vi "Configuration_table.vi"(11 "Configuration Queue":refnum<queue>) -> ()   [LabVIEW 2013, in "main.lvlib"]
uses:
  main.lvlib
  Controls/Reference AE Control.ctl
  Controls/Reference Cluster.ctl
  Bluetooth/MessageStructure.ctl
panel:
  in  "ActivityBox":bool caption="Efter stimulering"
  out "SegmentNumberString":string caption="Nummer"
  out "UndersøgelsesString":string caption="Undersøgelse"
  in  "ListboxLeftSegmentNr":i32(listbox) caption="Venstre"
  in  "ListboxRightSegmentNr":i32(listbox) caption="Højre"
  in  "ListboxMeasurementArea":i32(listbox) caption="Segment"
  in  "ListboxMeasurementTechnique":i32(listbox) caption="Teknik"
  in  "ListboxMeasurementMeth":i32(listbox) caption="Metode"
  out "Left Time Table":string[][](table)
  out "LeftArmPressureTable":string[][](table)
  out "LeftArmPulsTable":string[][](table)
  out "Right Time Table":string[][](table)
  out "RightArmPressureTable":string[][](table)
  out "RightArmPulsTable":string[][](table)
  in  "EditPressureBtn":bool
  in  "AddNewMeasurementBtn":bool
  in  "HeightAdjustmentInt":dbl caption="Højdejustering"
  in  "PalpationLeft":string(combo)="None" caption="Palpation"
  in  "PalpationRight":string(combo)="None" caption="Palpation"
  in  "Stop":bool
  # "Venstre"
  # "Sys"
  # "Dia"
  # "Puls"
  # "Tid"
  # "Højre"
  # "Tid"
  # "Sys"
  # "Dia"
  # "Puls"
  # "Palpation"
  # "cm"
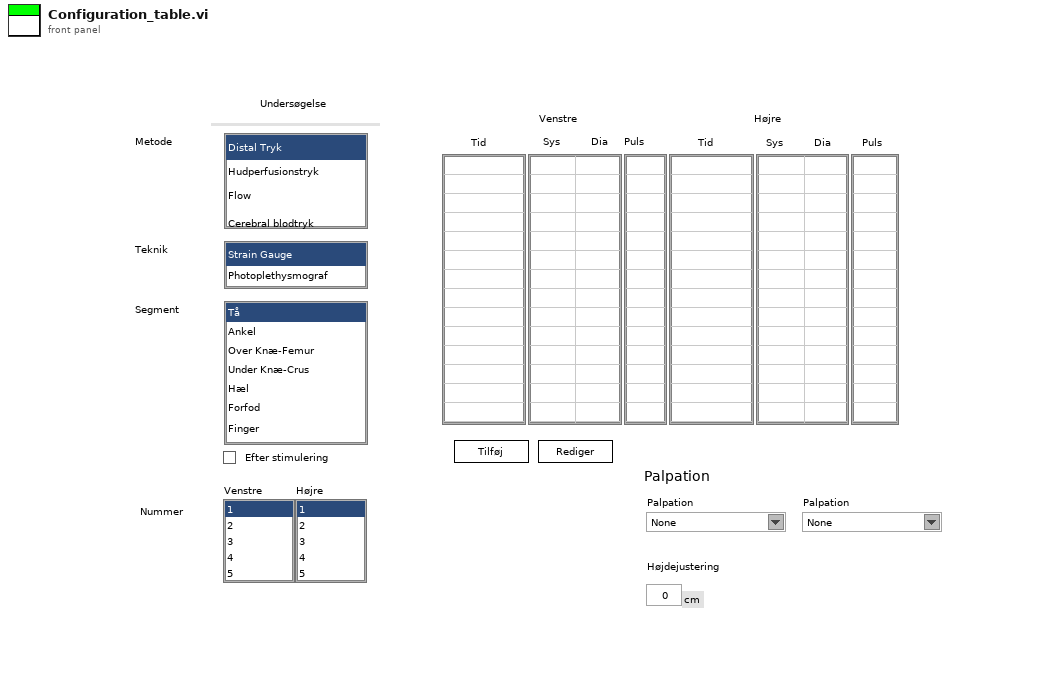
[diagram p1: front panel]
types:
  T1 = cluster{"sys":dbl, "dia":dbl, "puls":dbl, "date":string, "time":string, "code":string, "serial":string, "temp":dbl, "activity":string}
  T2 = typedef "main.lvlib/Reference AE Control.ctl" = enum16{"Initialize", "Set Menu", "Set Profile", "Set Configuration", "Set Configuration_old", "Set Configuration_new", "Set Configuration Method", "Set Acquisition", "Set Data", "Set Journal", "Get"}
  T3 = typedef "main.lvlib/Reference Cluster.ctl" = cluster{"Menu":cluster{"References":cluster{"Stop Acq":refnum<vi>, "MenuExit":refnum<vi>, "MenuStartADC":refnum<vi>, "PersonalInfoString":refnum<vi>, "Profile":refnum<vi>, "Configuration":refnum<vi>, "Acquisition":refnum<vi>, "Data":refnum<vi>, "Journal":refnum<vi>}}, "Profile":cluster{"References":cluster{"Search Patient ID":refnum<vi>, "Name":refnum<vi>, "CommentStr":refnum<vi>, "Listbox Patient ID":refnum<vi>, "ListboxDoctor":refnum<vi>, "ListboxOperator":refnum<vi>, "HospitalName":refnum<vi>, "HospitalDepartment":refnum<vi>, "HospitalAddress":refnum<vi>, "EditHospInfo":refnum<vi>, "Add Patient ID Btn":refnum<vi>, "Query Worklist":refnum<vi>}}, "Configuration":cluster{"References":cluster{"ListboxMeasurementArea":refnum<vi>, "ListboxMeasurementTechnique":refnum<vi>, "ListboxMeasurementMeth":refnum<vi>, "ListboxRightSegmentNr":refnum<vi>, "ListboxLeftSegmentNr":refnum<vi>, "HeightAdjustmentInt":refnum<vi>, "PalpationRight":refnum<vi>, "PalpationLeft":refnum<vi>, "ActivityBox":refnum<vi>}, "New method":cluster{"AddNewMeasurementBtn":refnum<vi>, "Left Time Table":refnum<vi>, "Right Time Table":refnum<vi>}, "Old method":cluster{"LeftArmPressureTable":refnum<vi>, "RightArmPressureTable":refnum<vi>, "SaveArmPressureBtn":refnum<vi>, "Puls":refnum<vi>, "TempTwo":refnum<vi>, "TempOne":refnum<vi>}, "Method":string}, "Acquisition":cluster{"References":cluster{"SegmentAcqString":refnum<vi>, "RingActGraph":refnum<vi>}}, "Data":cluster{"References":cluster{"cmString":refnum<vi>, "AdjustedHeight":refnum<vi>, "Menu":refnum<vi>, "Tangent On/Off":refnum<vi>, "FilterControl":refnum<vi>}}, "Journal":cluster{"References":cluster{"ReportSelection":refnum<vi>, "Data":refnum<vi>, "GenerateReport":refnum<vi>, "Menu":refnum<vi>, "Send To PACS":refnum<vi>}}}
  T4 = cluster{"ListboxMeasurementArea":refnum<vi>, "ListboxMeasurementTechnique":refnum<vi>, "ListboxMeasurementMeth":refnum<vi>, "ListboxRightSegmentNr":refnum<vi>, "ListboxLeftSegmentNr":refnum<vi>, "HeightAdjustmentInt":refnum<vi>, "PalpationRight":refnum<vi>, "PalpationLeft":refnum<vi>, "ActivityBox":refnum<vi>}
  T5 = typedef "LVRectTypeDef.ctl" = cluster{"Left":i16, "Top":i16, "Right":i16, "Bottom":i16}
  T6 = cluster{"ArmPressureSys":dbl, "ArmPressureDia":dbl, "ArmPuls":dbl, "Side":string}
  T7 = typedef "main.lvlib/MessageStructure.ctl" = cluster{"Type":i32, "Device type":i32, "Date":string, "Time":string, "Serial Number":string, "Sys":i32, "Dia":i32, "Puls":i32, "MAP":i32, "Code":string}
  T8 = cluster{"data":cluster{"sys":dbl, "dia":dbl, "puls":dbl, "date":string, "time":string, "code":string, "serial":string, "temp":dbl, "activity":string}, "Side":string}
  T9 = cluster{"sys":dbl, "dia":dbl, "puls":dbl, "date":string, "time":string, "code":string, "serial":string, "temp":dbl, "activity":string}[]
  T10 = cluster{"data":cluster{"sys":dbl, "dia":dbl, "puls":dbl, "date":string, "time":string, "code":string, "serial":string, "temp":dbl, "activity":string}, string}
  T11 = cluster{"AddNewMeasurementBtn":refnum<vi>, "Left Time Table":refnum<vi>, "Right Time Table":refnum<vi>}
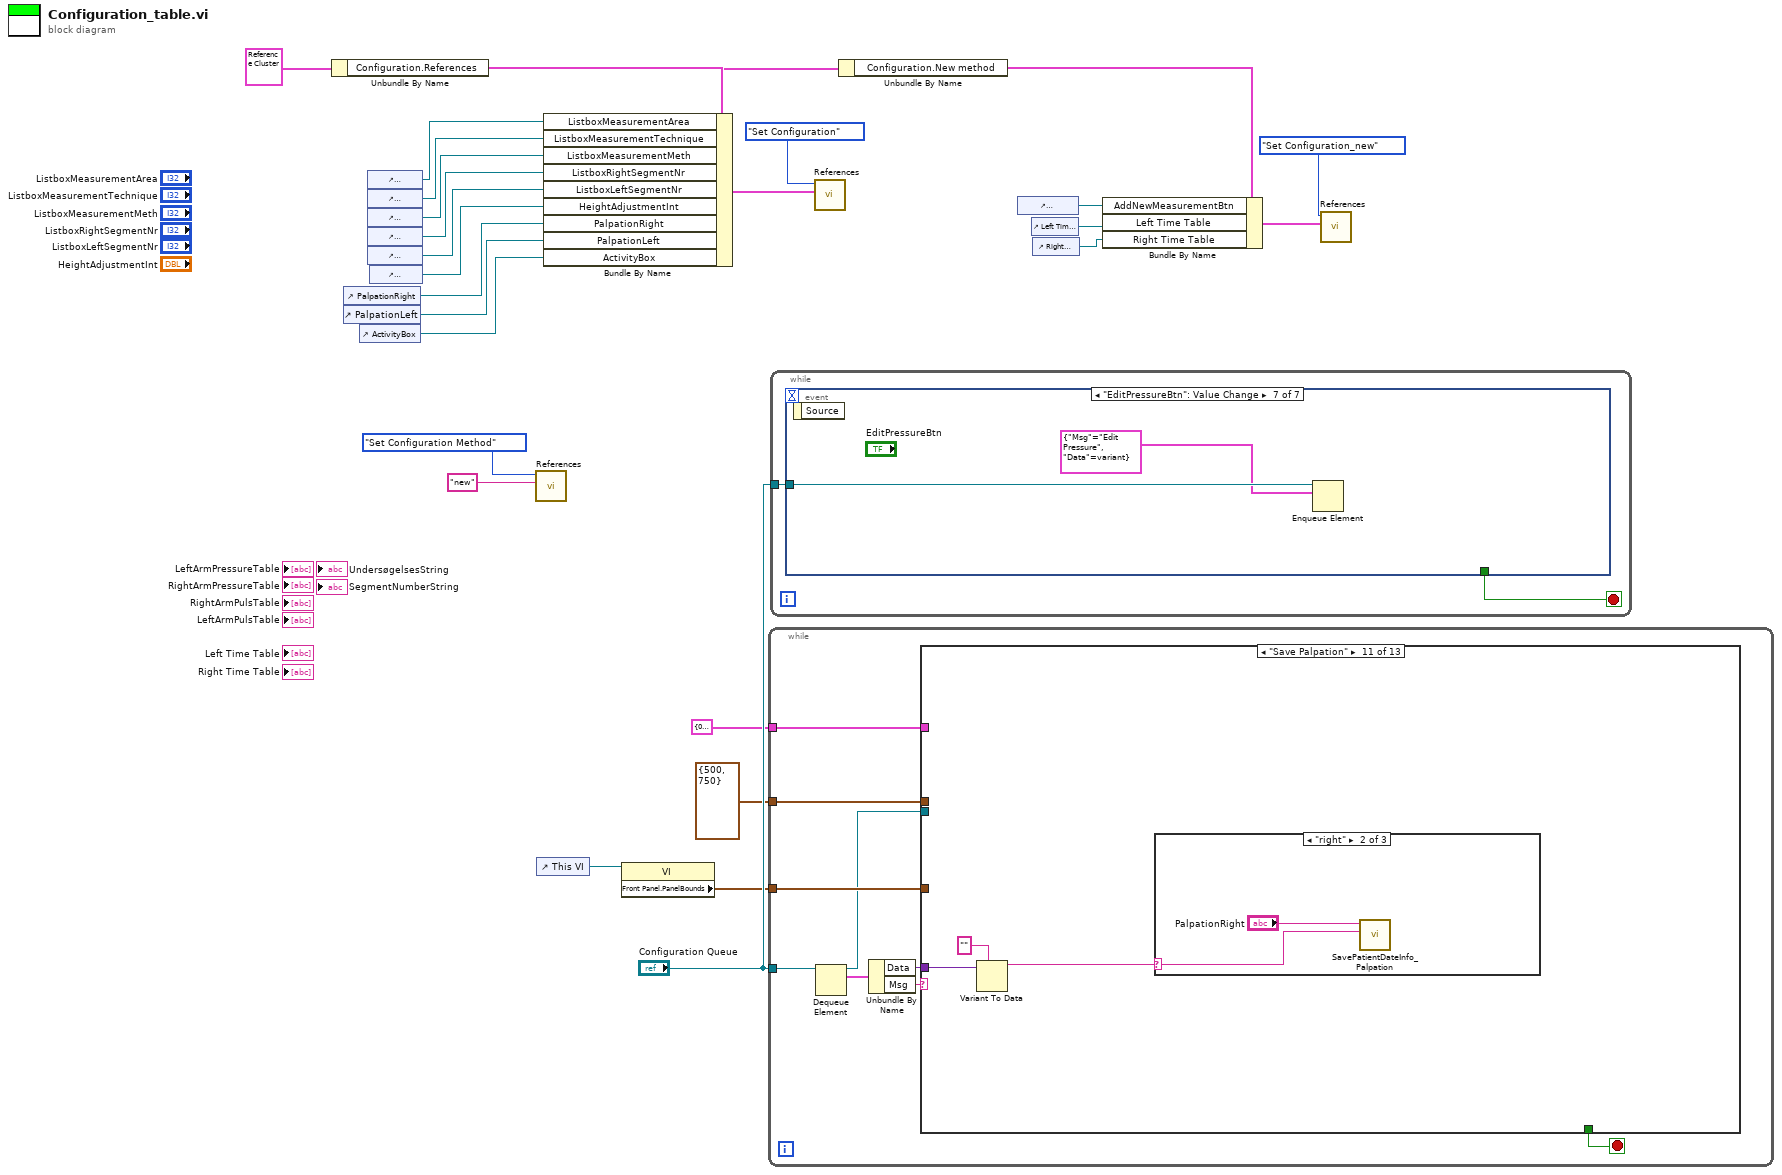
[diagram p0: block diagram]
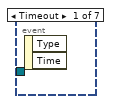
[diagram p2: hidden frame]
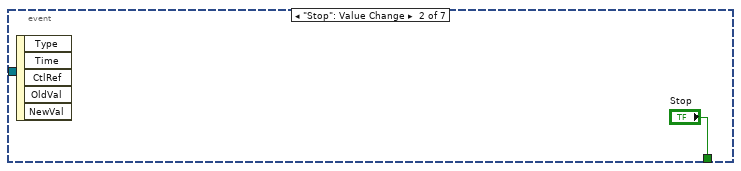
[diagram p3: hidden frame]
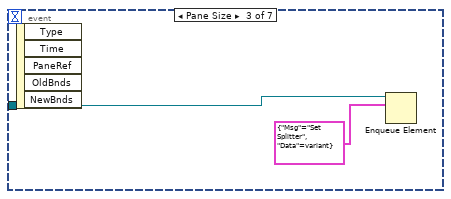
[diagram p4: hidden frame]
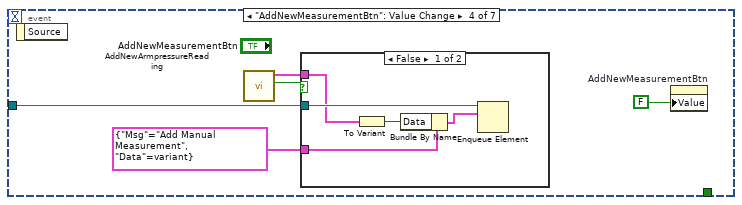
[diagram p5: hidden frame]
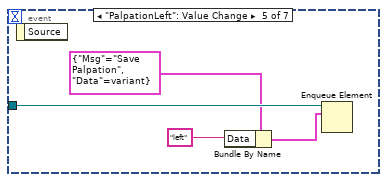
[diagram p7: hidden frame]
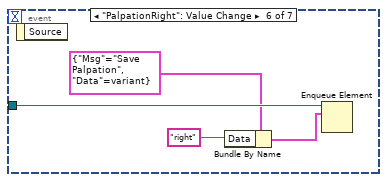
[diagram p8: hidden frame]
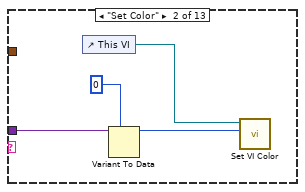
[diagram p10: hidden frame]
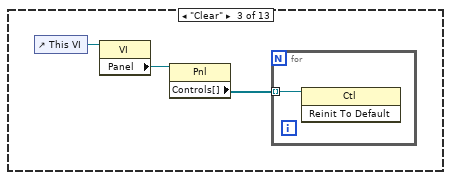
[diagram p11: hidden frame]
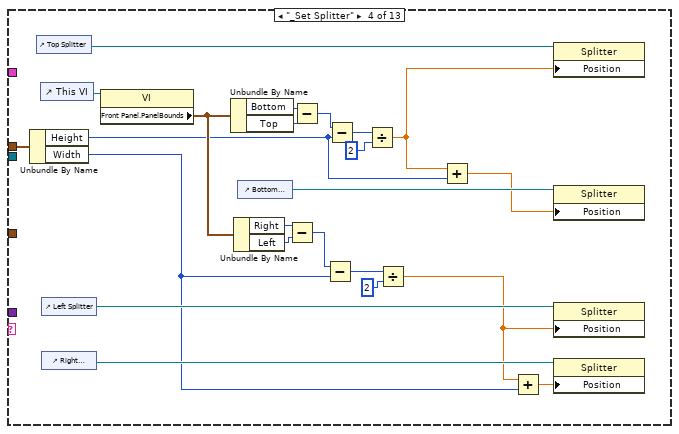
[diagram p12: hidden frame]
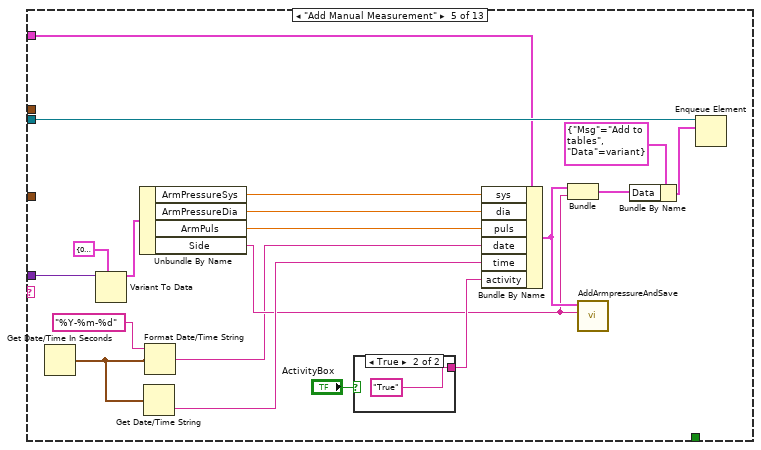
[diagram p13: hidden frame]
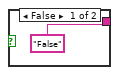
[diagram p14: hidden frame]
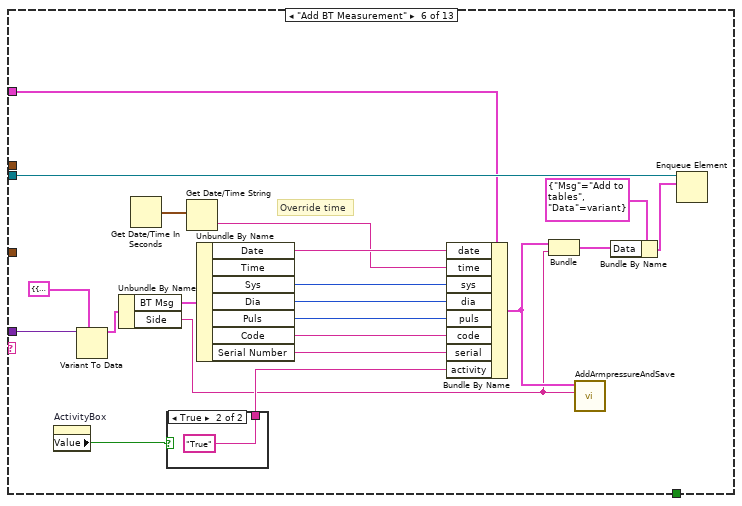
[diagram p15: hidden frame]
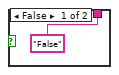
[diagram p16: hidden frame]
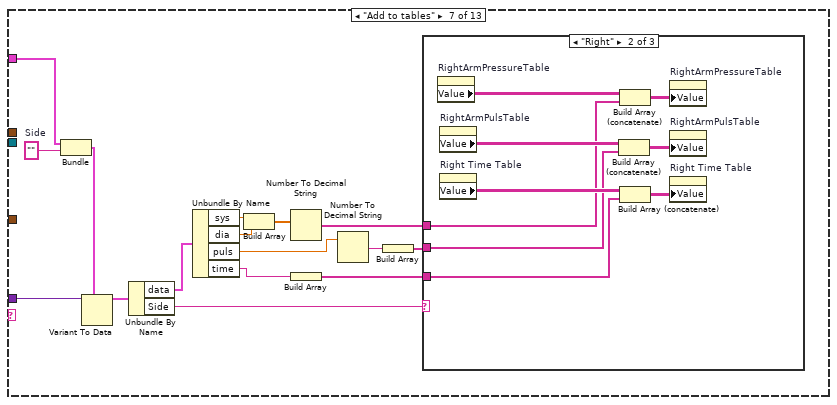
[diagram p17: hidden frame]
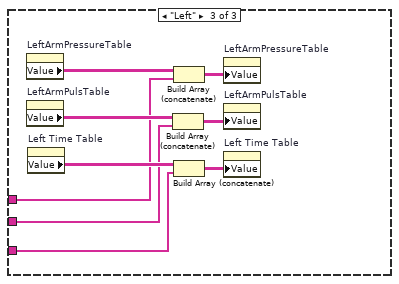
[diagram p19: hidden frame]
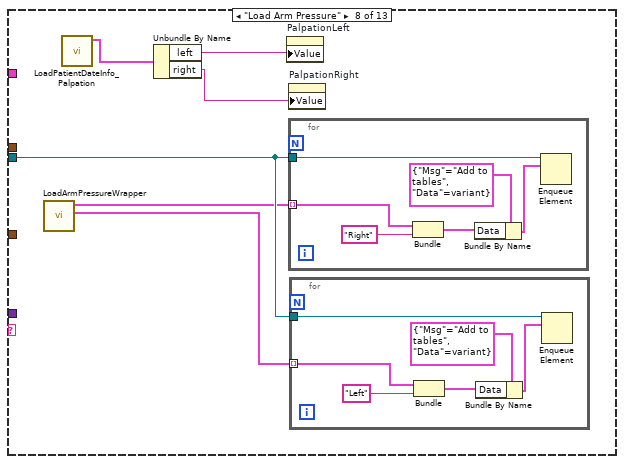
[diagram p20: hidden frame]
diagram:
  w10 = T3 {"Menu"={"References"={"Stop Acq"=refnum, "MenuExit"=refnum, "MenuStartADC"=refnum, "PersonalInfoString"=refnum, "Profile"=refnum, "Configuration"=refnum, "Acquisition"=refnum, "Data"=refnum, "Journal"=refnum}}, "Profile"={"References"={"Search Patient ID"=refnum, "Name"=refnum, "CommentStr"=refnum, "Listbox Patient ID"=refnum, "ListboxDoctor"=refnum, "ListboxOperator"=refnum, "HospitalName"=refnum, "HospitalDepartment"=refnum, "HospitalAddress"=refnum, "EditHospInfo"=refnum, "Add Patient ID Btn"=refnum, "Query Worklist"=refnum}}, "Configuration"={"References"={"ListboxMeasurementArea"=refnum, "ListboxMeasurementTechnique"=refnum, "ListboxMeasurementMeth"=refnum, "ListboxRightSegmentNr"=refnum, "ListboxLeftSegmentNr"=refnum, "HeightAdjustmentInt"=refnum, "PalpationRight"=refnum, "PalpationLeft"=refnum, "ActivityBox"=refnum}, "New method"={"AddNewMeasurementBtn"=refnum, "Left Time Table"=refnum, "Right Time Table"=refnum}, "Old method"={"LeftArmPressureTable"=refnum, "RightArmPressureTable"=refnum, "SaveArmPressureBtn"=refnum, "Puls"=refnum, "TempTwo"=refnum, "TempOne"=refnum}, "Method"=""}, "Acquisition"={"References"={"SegmentAcqString"=refnum, "RingActGraph"=refnum}}, "Data"={"References"={"cmString"=refnum, "AdjustedHeight"=refnum, "Menu"=refnum, "Tangent On/Off"=refnum, "FilterControl"=refnum}}, "Journal"={"References"={"ReportSelection"=refnum, "Data"=refnum, "GenerateReport"=refnum, "Menu"=refnum, "Send To PACS"=refnum}}}
  n1 = Unbundle By Name(w10) -> ("Configuration.References"=w11:T4)
  n2 = control-ref of="PalpationRight"() -> (w14:refnum<vi>)
  n3 = control-ref of="PalpationLeft"() -> (w13:refnum<vi>)
  n4 = control-ref of="ActivityBox"() -> (w12:refnum<vi>)
  n5 = control-ref of="ListboxMeasurementArea"() -> (w26:refnum<vi>)
  n6 = control-ref of="ListboxMeasurementTechnique"() -> (w25:refnum<vi>)
  n7 = control-ref of="ListboxMeasurementMeth"() -> (w24:refnum<vi>)
  n8 = control-ref of="ListboxRightSegmentNr"() -> (w23:refnum<vi>)
  n9 = control-ref of="ListboxLeftSegmentNr"() -> (w22:refnum<vi>)
  n10 = control-ref of="HeightAdjustmentInt"() -> (w21:refnum<vi>)
  n11 = call "References.vi"("variant"="new", "Reference AE Control"=Reference_AE_Control."Set Configuration Method") -> ()  [unwired: 8 in, 2 out]
  n12 = control-ref of="This VI"() -> (w17:refnum<vi>)
  n13 = Bundle By Name(cluster=w11, "ListboxMeasurementArea"=w26, "ListboxMeasurementTechnique"=w25, "ListboxMeasurementMeth"=w24, "ListboxRightSegmentNr"=w23, "ListboxLeftSegmentNr"=w22, "HeightAdjustmentInt"=w21, "PalpationRight"=w14, "PalpationLeft"=w13, "ActivityBox"=w12) -> (w19:T4)
  n14 = property class="VI"(reference=w17) -> ("Front Panel.PanelBounds"=w16:T5)  [unwired: 1 in, 2 out]
  n15 = while {
    tunnel: "Configuration Queue" -> [w35]
    tunnel: cluster{"Height":i32, "Width":i32} {"Height"=500, "Width"=750} -> [w30]
    tunnel: w16 -> [w29]
    tunnel: T1 {"sys"=0.0, "dia"=0.0, "puls"=0.0, "date"="", "time"="", "code"="", "serial"="", "temp"=0.0, "activity"=""} ("data") -> [w27]
    stop <- w32 stop-if-true
    n16 = Dequeue Element(queue=w35) -> (queue out=w28:refnum<queue>, element=w34:cluster{"Msg":string, "Data":variant})  [unwired: 2 in, 2 out]
    n17 = Unbundle By Name(w34) -> ("Data"=w31:variant, "Msg"=w33:string)
    n18 = case shown="\"Save Palpation\"" w33 {
      tunnel: [_ _ _ _ _ _ _ _ _ _ _ w185 w207] -> w32
      tunnel: w31 -> [_ w36 _ _ w85 w108 w126 _ _ _ w179 _ _]
      tunnel: w30 -> [_ _ _ w52 _ _ _ _ _ _ _ w194 _]
      tunnel: w29 -> [_ _ _ _ _ _ _ _ _ _ _ w184 _]
      tunnel: w28 -> [_ _ _ _ w81 w106 _ w150 w163 _ _ _ _]
      tunnel: w27 -> [_ _ _ _ w76 w93 w122 _ _ _ _ _ _]
      frame "", Default {
      }
      frame "Set Color" {
        n19 = control-ref of="This VI"() -> (w39:refnum<vi>)
        n20 = Variant To Data(type=u32 0 ("Pane Color"), Variant=w36) -> (data=w37:u32)  [unwired: 1 in, 1 out]
        n21 = call "Set VI Color.vi"("Pane Color"=w37, "VI in"=w39) -> ()  [unwired: 10 in]
      }
      frame "Clear" {
        n22 = control-ref of="This VI"() -> (w42:refnum<vi>)
        n23 = property class="VI"(reference=w42) -> ("Panel"=w41:refnum<vi>)  [unwired: 1 in, 2 out]
        n24 = property class="Pnl"(reference=w41) -> ("Controls[]"=w40:refnum<vi>[])  [unwired: 1 in, 2 out]
        n25 = for {
          tunnel: w40 -> [w43] mode=indexing
          n26 = invoke class="Ctl" method="Reinit To Default"(reference=w43) -> ()  [unwired: 2 in, 3 out]
        }
      }
      frame "_Set Splitter" {
        n27 = Unbundle By Name(w52) -> ("Height"=w50:i32, "Width"=w45:i32)
        n28 = control-ref of="Top Splitter"() -> (w60:refnum<vi>)
        n29 = control-ref of="This VI"() -> (w66:refnum<vi>)
        n30 = control-ref of="Left Splitter"() -> (w53:refnum<vi>)
        n31 = control-ref of="Right Splitter"() -> (w47:refnum<vi>)
        n32 = property class="VI"(reference=w66) -> ("Front Panel.PanelBounds"=w59:T5)  [unwired: 1 in, 2 out]
        n33 = Unbundle By Name(w59) -> ("Bottom"=w65:i16, "Top"=w64:i16)
        n34 = Unbundle By Name(w59) -> ("Right"=w58:i16, "Left"=w57:i16)
        n35 = control-ref of="Bottom Splitter"() -> (w49:refnum<vi>)
        n36 = Subtract(x=w58, y=w57) -> (x-y=w56:i16)
        n37 = Subtract(x=w65, y=w64) -> (x-y=w63:i16)
        n38 = Subtract(x=w56, y=w45) -> (x-y=w55:i32)
        n39 = Subtract(x=w63, y=w50) -> (x-y=w62:i32)
        n40 = Divide(x=w62, y=2) -> (x/y=w51:dbl)
        n41 = Divide(x=w55, y=u32 2) -> (x/y=w46:dbl)
        n42 = Add(x=w51, y=w50) -> (x+y=w48:dbl)
        n43 = Add(x=w46, y=w45) -> (x+y=w44:dbl)
        n44 = property class="Splitter"(reference=w60, "Position"=w51) -> ()  [unwired: 1 in, 2 out]
        n45 = property class="Splitter"(reference=w49, "Position"=w48) -> ()  [unwired: 1 in, 2 out]
        n46 = property class="Splitter"(reference=w53, "Position"=w46) -> ()  [unwired: 1 in, 2 out]
        n47 = property class="Splitter"(reference=w47, "Position"=w44) -> ()  [unwired: 1 in, 2 out]
      }
      frame "Add Manual Measurement" {
        n48 = Get Date/Time In Seconds() -> (seconds since 1Jan1904=w68:timestamp)
        n49 = Variant To Data(type=T6 {"ArmPressureSys"=0.0, "ArmPressureDia"=0.0, "ArmPuls"=0.0, "Side"=""} ("output cluster"), Variant=w85) -> (data=w74:T6)  [unwired: 1 in, 1 out]
        n50 = Unbundle By Name(w74) -> ("ArmPressureSys"=w73:dbl, "ArmPressureDia"=w72:dbl, "ArmPuls"=w71:dbl, "Side"=w70:string)
        n51 = Get Date/Time String(seconds (now)=w68) -> (time string=w84:string)  [unwired: 2 in, 1 out]
        n52 = Format Date/Time String(time format string (%c)="%Y-%m-%d", seconds (now)=w68) -> (date/time string=w67:string)  [unwired: 1 in]
        n53 = case shown="True" "ActivityBox" {
          tunnel: ["False" "True"] -> w82
          frame False {
          }
          frame True {
          }
        }
        n54 = Bundle By Name(cluster=w76, "sys"=w73, "dia"=w72, "puls"=w71, "date"=w67, "time"=w84, "activity"=w82) -> (w77:T1)
        n55 = Bundle("data"=w77, "Side"=w70) -> (w78:T8)  [unwired: 1 in]
        n56 = call "AddArmpressureAndSave.vi"("Side(Left/Right)"=w70, "data"=w77) -> ()  [unwired: 9 in, 1 out]
        n57 = Bundle By Name(cluster=cluster{"Msg":string, "Data":variant} {"Msg"="Add to tables", "Data"=variant} ("element"), "Data"=w78) -> (w79:cluster{"Msg":string, "Data":variant})
        n58 = Enqueue Element(queue=w81, element=w79) -> ()  [unwired: 2 in, 3 out]
      }
      frame "Add BT Measurement" {
        # "Override time"
        n59 = property on="ActivityBox" class="Bool (strict)"() -> ("Value"=w94:bool)  [unwired: 2 in, 2 out]
        n60 = Variant To Data(type=cluster{"BT Msg":T7, "Side":string} {"BT Msg"={"Type"=0, "Device type"=0, "Date"="", "Time"="", "Serial Number"="", "Sys"=0, "Dia"=0, "Puls"=0, "MAP"=0, "Code"=""}, "Side"=""}, Variant=w108) -> (data=w97:cluster{"BT Msg":T7, "Side":string})  [unwired: 1 in, 1 out]
        n61 = Unbundle By Name(w97) -> ("BT Msg"=w96:T7, "Side"=w95:string)
        n62 = Get Date/Time In Seconds() -> (seconds since 1Jan1904=w89:timestamp)
        n63 = case shown="True" w94 {
          tunnel: ["False" "True"] -> w107
          frame False {
          }
          frame True {
          }
        }
        n64 = Get Date/Time String(seconds (now)=w89) -> (time string=w88:string)  [unwired: 2 in, 1 out]
        n65 = Unbundle By Name(w96) -> ("Date"=w91:string, "Sys"=w92:i32, "Dia"=w101:i32, "Puls"=w100:i32, "Code"=w99:string, "Serial Number"=w98:string)  [unwired: 1 out]
        n66 = Bundle By Name(cluster=w93, "date"=w91, "time"=w88, "sys"=w92, "dia"=w101, "puls"=w100, "code"=w99, "serial"=w98, "activity"=w107) -> (w102:T1)
        n67 = Bundle("data"=w102, "Side"=w95) -> (w103:T8)  [unwired: 1 in]
        n68 = call "AddArmpressureAndSave.vi"("Side(Left/Right)"=w95, "data"=w102) -> ()  [unwired: 9 in, 1 out]
        n69 = Bundle By Name(cluster=cluster{"Msg":string, "Data":variant} {"Msg"="Add to tables", "Data"=variant} ("element"), "Data"=w103) -> (w104:cluster{"Msg":string, "Data":variant})
        n70 = Enqueue Element(queue=w106, element=w104) -> ()  [unwired: 2 in, 3 out]
      }
      frame "Add to tables" {
        w123 = ""  # Side
        n71 = Bundle("data"=w122, "Side"=w123) -> (w121:T8)  [unwired: 1 in]
        n72 = Variant To Data(type=w121, Variant=w126) -> (data=w125:T8)  [unwired: 1 in, 1 out]
        n73 = Unbundle By Name(w125) -> ("data"=w118:T1, "Side"=w124:string)
        n74 = Unbundle By Name(w118) -> ("sys"=w119:dbl, "dia"=w120:dbl, "puls"=w114:dbl, "time"=w111:string)
        n75 = Build Array(w119, w120) -> (w117:dbl[])
        n76 = Number To Decimal String(number=w117) -> (decimal integer string=w116:string[])  [unwired: 1 in]
        n77 = Build Array(w111) -> (w115:string[])
        n78 = Number To Decimal String(number=w114) -> (decimal integer string=w112:string)  [unwired: 1 in]
        n79 = Build Array(w112) -> (w113:string[])
        n80 = case shown="\"Right\"" w124 {
          tunnel: w113 -> [_ w129 w138]
          tunnel: w116 -> [_ w128 w137]
          tunnel: w115 -> [_ w127 w136]
          frame "False", Default {
          }
          frame "Right" {
            n81 = property on="RightArmPressureTable" class="Tbl (strict)"() -> ("Value"=w135:string[][])  [unwired: 2 in, 2 out]
            n82 = property on="RightArmPulsTable" class="Tbl (strict)"() -> ("Value"=w132:string[][])  [unwired: 2 in, 2 out]
            n83 = property on="Right Time Table" class="Tbl (strict)"() -> ("Value"=w131:string[][])  [unwired: 2 in, 2 out]
            n84 = Build Array (concatenate)(w132, w129) -> (w133:string[][])
            n85 = Build Array (concatenate)(w135, w128) -> (w134:string[][])
            n86 = Build Array (concatenate)(w131, w127) -> (w130:string[][])
            n87 = property on="RightArmPressureTable" class="Tbl (strict)"("Value"=w134) -> ()  [unwired: 2 in, 2 out]
            n88 = property on="RightArmPulsTable" class="Tbl (strict)"("Value"=w133) -> ()  [unwired: 2 in, 2 out]
            n89 = property on="Right Time Table" class="Tbl (strict)"("Value"=w130) -> ()  [unwired: 2 in, 2 out]
          }
          frame "Left" {
            n90 = property on="LeftArmPressureTable" class="Tbl (strict)"() -> ("Value"=w144:string[][])  [unwired: 2 in, 2 out]
            n91 = property on="LeftArmPulsTable" class="Tbl (strict)"() -> ("Value"=w143:string[][])  [unwired: 2 in, 2 out]
            n92 = property on="Left Time Table" class="Tbl (strict)"() -> ("Value"=w142:string[][])  [unwired: 2 in, 2 out]
            n93 = Build Array (concatenate)(w143, w138) -> (w140:string[][])
            n94 = Build Array (concatenate)(w144, w137) -> (w141:string[][])
            n95 = Build Array (concatenate)(w142, w136) -> (w139:string[][])
            n96 = property on="LeftArmPressureTable" class="Tbl (strict)"("Value"=w141) -> ()  [unwired: 2 in, 2 out]
            n97 = property on="LeftArmPulsTable" class="Tbl (strict)"("Value"=w140) -> ()  [unwired: 2 in, 2 out]
            n98 = property on="Left Time Table" class="Tbl (strict)"("Value"=w139) -> ()  [unwired: 2 in, 2 out]
          }
        }
      }
      frame "Load Arm Pressure" {
        n99 = call "LoadArmPressureWrapper.vi"() -> ("Armpressure Left"=w145:T9, "Armpressure Right"=w146:T9)  [unwired: 9 in, 1 out]
        n100 = call "LoadPatientDateInfo_Palpation.vi"() -> ("palpation"=w147:cluster{"right":string, "left":string})  [unwired: 10 in, 1 out]
        n101 = Unbundle By Name(w147) -> ("left"=w149:string, "right"=w148:string)
        n102 = property on="PalpationLeft" class="CmbBox"("Value"=w149) -> ()  [unwired: 2 in, 2 out]
        n103 = property on="PalpationRight" class="CmbBox"("Value"=w148) -> ()  [unwired: 2 in, 2 out]
        n104 = for {
          tunnel: w150 -> [w159]
          tunnel: w146 -> [w158] mode=indexing
          n105 = Bundle("data"=w158, "Right") -> (w160:T10)  [unwired: 1 in]
          n106 = Bundle By Name(cluster=cluster{"Msg":string, "Data":variant} {"Msg"="Add to tables", "Data"=variant} ("element"), "Data"=w160) -> (w161:cluster{"Msg":string, "Data":variant})
          n107 = Enqueue Element(queue=w159, element=w161) -> ()  [unwired: 2 in, 3 out]
        }
        n108 = for {
          tunnel: w150 -> [w153]
          tunnel: w145 -> [w152] mode=indexing
          n109 = Bundle("data"=w152, "Left") -> (w154:T10)  [unwired: 1 in]
          n110 = Bundle By Name(cluster=cluster{"Msg":string, "Data":variant} {"Msg"="Add to tables", "Data"=variant} ("element"), "Data"=w154) -> (w155:cluster{"Msg":string, "Data":variant})
          n111 = Enqueue Element(queue=w153, element=w155) -> ()  [unwired: 2 in, 3 out]
        }
      }
      frame "Edit Pressure" {
        n112 = call "EditPatientDataInfoArmPressure.vi"() -> ("Save?"=w164:bool)  [unwired: 11 in]
        n113 = case shown="True" w164 {
          tunnel: w163 -> [_ w167]
          frame False {
          }
          frame True {
            # "Update UI"
            n114 = Enqueue Element(queue=w167, element=cluster{"Msg":string, "Data":variant} {"Msg"="Clear Pressure Tables", "Data"=variant}) -> (queue out=w166:refnum<queue>)  [unwired: 2 in, 2 out]
            n115 = Enqueue Element(queue=w166, element=cluster{"Msg":string, "Data":variant} {"Msg"="Load Arm Pressure", "Data"=variant}) -> ()  [unwired: 2 in, 3 out]
          }
        }
      }
      frame "Clear Pressure Tables" {
        n116 = control-ref of="LeftArmPressureTable"() -> (w175:refnum<vi>)
        n117 = control-ref of="RightArmPressureTable"() -> (w174:refnum<vi>)
        n118 = control-ref of="RightArmPulsTable"() -> (w173:refnum<vi>)
        n119 = control-ref of="LeftArmPulsTable"() -> (w172:refnum<vi>)
        n120 = control-ref of="Left Time Table"() -> (w171:refnum<vi>)
        n121 = control-ref of="Right Time Table"() -> (w170:refnum<vi>)
        n122 = Build Array(w175, w174, w173, w172, w171, w170) -> (w169:refnum<vi>[])
        n123 = for {
          tunnel: w169 -> [w176] mode=indexing
          n124 = invoke class="Tbl (strict)" method="Reinit To Default"(reference=w176) -> ()  [unwired: 2 in, 3 out]
        }
      }
      frame "Save Palpation" {
        n125 = Variant To Data(type="", Variant=w179) -> (data=w177:string)  [unwired: 1 in, 1 out]
        n126 = case shown="\"right\"" w177 {
          selector: w177 -> [_ w180 w182]
          frame "False", Default {
          }
          frame "right" {
            n127 = call "SavePatientDateInfo_Palpation.vi"("side(left/right)"=w180, "palpation"="PalpationRight") -> ()  [unwired: 9 in, 1 out]
          }
          frame "left" {
            n128 = call "SavePatientDateInfo_Palpation.vi"("side(left/right)"=w182, "palpation"="PalpationLeft") -> ()  [unwired: 9 in, 1 out]
          }
        }
      }
      frame "_Stop" {
        w185 = TRUE
        n129 = Unbundle By Name(w194) -> ("Height"=w192:i32, "Width"=w187:i32)
        n130 = control-ref of="Top Splitter"() -> (w201:refnum<vi>)
        n131 = control-ref of="Left Splitter"() -> (w195:refnum<vi>)
        n132 = control-ref of="Right Splitter"() -> (w189:refnum<vi>)
        n133 = Unbundle By Name(w184) -> ("Bottom"=w206:i16, "Top"=w205:i16)
        n134 = Unbundle By Name(w184) -> ("Right"=w200:i16, "Left"=w199:i16)
        n135 = control-ref of="Bottom Splitter"() -> (w191:refnum<vi>)
        n136 = Subtract(x=w200, y=w199) -> (x-y=w198:i16)
        n137 = Subtract(x=w206, y=w205) -> (x-y=w204:i16)
        n138 = Subtract(x=w198, y=w187) -> (x-y=w197:i32)
        n139 = Subtract(x=w204, y=w192) -> (x-y=w203:i32)
        n140 = Divide(x=w203, y=2) -> (x/y=w193:dbl)
        n141 = Divide(x=w197, y=u32 2) -> (x/y=w188:dbl)
        n142 = Add(x=w193, y=w192) -> (x+y=w190:dbl)
        n143 = Add(x=w188, y=w187) -> (x+y=w186:dbl)
        n144 = property class="Splitter"(reference=w201, "Position"=w193) -> ()  [unwired: 1 in, 2 out]
        n145 = property class="Splitter"(reference=w191, "Position"=w190) -> ()  [unwired: 1 in, 2 out]
        n146 = property class="Splitter"(reference=w195, "Position"=w188) -> ()  [unwired: 1 in, 2 out]
        n147 = property class="Splitter"(reference=w189, "Position"=w186) -> ()  [unwired: 1 in, 2 out]
        n148 = property on="Stop" class="Bool (strict)"("Val(Sgnl)"=w185) -> ()  [unwired: 2 in, 2 out]
      }
      frame "Stop" {
        w207 = TRUE
        n149 = property on="Stop" class="Bool (strict)"("Val(Sgnl)"=w207) -> ()  [unwired: 2 in, 2 out]
      }
    }
  }
  n150 = while {
    tunnel: "Configuration Queue" -> [w209]
    stop <- w208 stop-if-true
    n151 = event shown="[6] \"EditPressureBtn\": Value Change" {
      selector: _ -> [_ _ _ _ _ _ _]
      dyn-events: _ -> [_ _ _ _ _ _ _]
      timeout: _ -> [_ _ _ _ _ _ _]
      tunnel: w209 -> [_ _ w212 w217 w226 w230 w232]
      tunnel: [_ "Stop" _ _ _ _ _] -> w208
      event Timeout {
        n152 = event-data() -> ()  [unwired: 1 in, 2 out]
      }
      event "Stop": Value Change {
        n153 = event-data() -> ()  [unwired: 1 in, 5 out]
      }
      event Pane Size {
        n154 = event-data() -> ()  [unwired: 1 in, 5 out]
        n155 = Enqueue Element(queue=w212, element=cluster{"Msg":string, "Data":variant} {"Msg"="Set Splitter", "Data"=variant}) -> ()  [unwired: 2 in, 3 out]
      }
      event "AddNewMeasurementBtn": Value Change {
        n156 = event-data() -> ()  [unwired: 1 in, 1 out]
        n157 = call "AddNewArmpressureReading.vi"() -> ("Cancel?"=w214:bool, "output cluster"=w215:T6)  [unwired: 10 in]
        n158 = case shown="False" w214 {
          tunnel: w217 -> [w222 _]
          tunnel: cluster{"Msg":string, "Data":variant} {"Msg"="Add Manual Measurement", "Data"=variant} ("element") -> [w221 _]
          tunnel: w215 -> [w218 _]
          frame False {
            n159 = To Variant(anything=w218) -> (Variant=w219:variant)
            n160 = Bundle By Name(cluster=w221, "Data"=w219) -> (w220:cluster{"Msg":string, "Data":variant})
            n161 = Enqueue Element(queue=w222, element=w220) -> ()  [unwired: 2 in, 3 out]
          }
          frame True {
          }
        }
        n162 = property on="AddNewMeasurementBtn" class="Bool (strict)"("Value"=FALSE) -> ()  [unwired: 2 in, 2 out]
      }
      event "PalpationLeft": Value Change {
        n163 = event-data() -> ()  [unwired: 1 in, 1 out]
        n164 = Bundle By Name(cluster=cluster{"Msg":string, "Data":variant} {"Msg"="Save Palpation", "Data"=variant} ("element"), "Data"="left") -> (w224:cluster{"Msg":string, "Data":variant})
        n165 = Enqueue Element(queue=w226, element=w224) -> ()  [unwired: 2 in, 3 out]
      }
      event "PalpationRight": Value Change {
        n166 = event-data() -> ()  [unwired: 1 in, 1 out]
        n167 = Bundle By Name(cluster=cluster{"Msg":string, "Data":variant} {"Msg"="Save Palpation", "Data"=variant} ("element"), "Data"="right") -> (w228:cluster{"Msg":string, "Data":variant})
        n168 = Enqueue Element(queue=w230, element=w228) -> ()  [unwired: 2 in, 3 out]
      }
      event "EditPressureBtn": Value Change {
        n169 = event-data() -> ()  [unwired: 1 in, 1 out]
        n170 = Enqueue Element(queue=w232, element=cluster{"Msg":string, "Data":variant} {"Msg"="Edit Pressure", "Data"=variant}) -> ()  [unwired: 2 in, 3 out]
      }
    }
  }
  n171 = call "References.vi"("variant"=w19, "Reference AE Control"=Reference_AE_Control."Set Configuration") -> ()  [unwired: 8 in, 2 out]
  n172 = Unbundle By Name(w10) -> ("Configuration.New method"=w9:T11)
  n173 = control-ref of="AddNewMeasurementBtn"() -> (w8:refnum<vi>)
  n174 = control-ref of="Left Time Table"() -> (w7:refnum<vi>)
  n175 = control-ref of="Right Time Table"() -> (w2:refnum<vi>)
  n176 = Bundle By Name(cluster=w9, "AddNewMeasurementBtn"=w8, "Left Time Table"=w7, "Right Time Table"=w2) -> (w6:T11)
  n177 = call "References.vi"("variant"=w6, "Reference AE Control"=Reference_AE_Control."Set Configuration_new") -> ()  [unwired: 8 in, 2 out]
